vi "init_machine_state.vi"(2 "protocol":u16(ring) items=["None", "XON/XOFF", "RTS/CTS", "XON/XOFF & RTS/CTS", "DTR/DSR", "XON/XOFF & DTR/DSR"], 3 "COM":refnum<visa-resource-name>) -> (1 "output_machine_reference.lvclass":refnum<class "machine.lvclass">)   [LabVIEW 2014, in "machine.lvclass"]
uses:
  machine.lvclass
  machine.lvclass/machine.ctl
  <vilib>/Instr/_visa.llb/VISA Configure Serial Port (Instr).vi
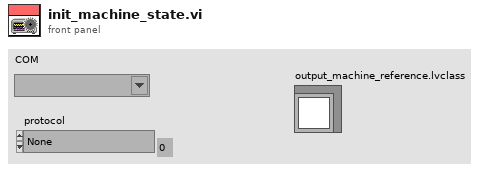
[diagram p1: front panel]
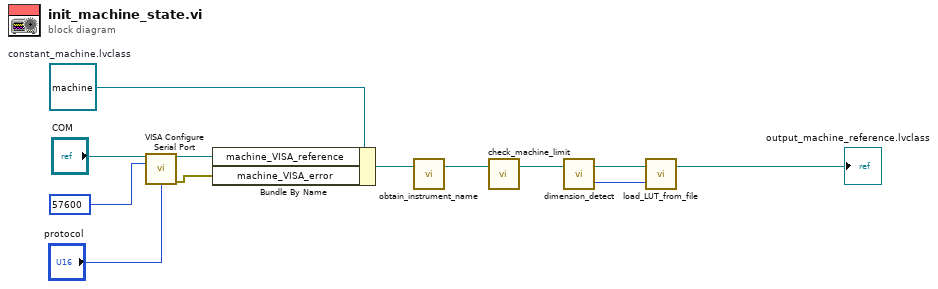
[diagram p0: block diagram]
diagram:
  w9 = refnum<class "machine.lvclass"> refnum  # constant_machine.lvclass
  n1 = call-poly "VISA Configure Serial Port"("VISA resource name"="COM", "baud rate (9600)"=u32 57600, "flow control (0:none)"="protocol") -> ("VISA resource name out"=w8:refnum<visa-resource-name>, "error out"=w7:errorcluster)  [unwired: 11 in]
  n2 = Bundle By Name(cluster=w9, "machine_VISA_reference"=w8, "machine_VISA_error"=w7) -> (w6:refnum<class "machine.lvclass">)
  n3 = call "obtain_instrument_name.vi"("input_machine_reference.lvclass"=w6) -> ("output_machine_reference.lvclass"=w5:refnum<class "machine.lvclass">)  [unwired: 2 in]
  n4 = call "check_machine_limit.vi"("input_machine_reference.lvclass"=w5) -> ("output_machine_reference.lvclass"=w4:refnum<class "machine.lvclass">)  [unwired: 2 in]
  n5 = call "dimension_detect.vi"("input_machine_reference.lvclass"=w4) -> ("SCPI_comand_array_size"=w2:u32, "output_machine_reference.lvclass"=w3:refnum<class "machine.lvclass">)  [unwired: 1 in]
  n6 = call "load_LUT_from_file.vi"("command_array_length"=w2, "input_machine_reference.lvclass"=w3) -> ("output_machine_reference.lvclass"=→"output_machine_reference.lvclass":refnum<class "machine.lvclass">)  [unwired: 1 in]
